vi "Get Enabled Measurements.vi"(8 "error in (no error)":errorcluster, 11 "Cluster in":T1) -> (0 "error out":errorcluster, 3 "Enabled Measurements":bool[](array[boolean]))   [LabVIEW 2019, in "ZenGage v3.0 UI.lvclass"]
uses:
  ZenGage v3.0 UI.lvclass
  <vilib>/Utility/miscctls.llb/LVRowAndColumnTypeDef.ctl
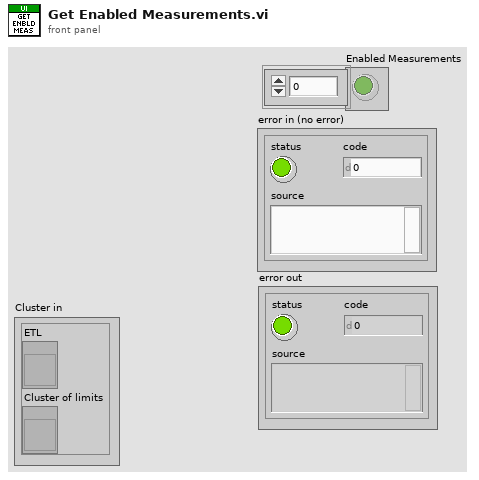
[diagram p1: front panel]
types:
  T1 = cluster{"ETL":refnum<vi>, "Cluster of limits":refnum<vi>}
  T2 = enum8{"Enabled", "Disabled", "Disabled and Grayed Out"}
  T3 = typedef "LVRowAndColumnTypeDef.ctl" = cluster{"Row":i32, "Column":i32}
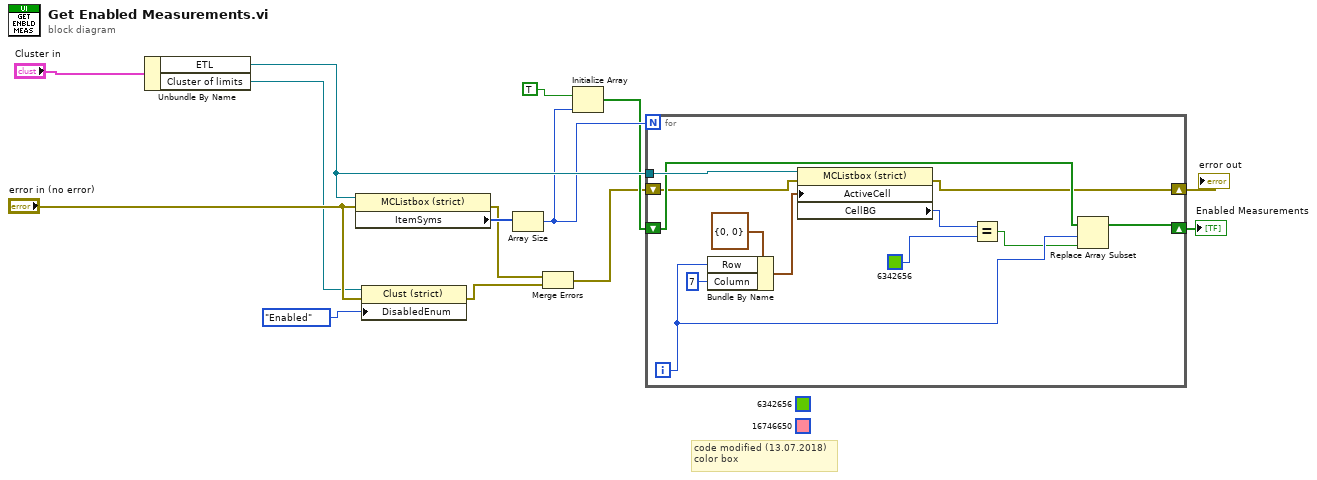
[diagram p0: block diagram]
diagram:
  (unwired) u32 6342656
  (unwired) u32 16746650
  # "code modified (13.07.2018)\ncolor box"
  n1 = Unbundle By Name("Cluster in") -> ("ETL"=w13:refnum<vi>, "Cluster of limits"=w4:refnum<vi>)
  n2 = property class="MCListbox (strict)"(reference=w13, error in="error in (no error)") -> (error out=w2:errorcluster, "ItemSyms"=w12:i32[])  [unwired: 1 out]
  n3 = property class="Clust (strict)"(reference=w4, error in="error in (no error)", "DisabledEnum"=T2."Enabled" ("Disabled")) -> (error out=w3:errorcluster)  [unwired: 1 out]
  n4 = Array Size(array=w12) -> (size(s)=w10:i32)
  n5 = Merge Errors(w2, w3) -> (w1:errorcluster)
  n6 = Initialize Array(TRUE, w10) -> (w9:bool[])
  n7 = for {
    N: w10 -> [_]
    tunnel: w13 -> [w26]
    shift-right: [w18] -> w8
    shift-left: w9 -> [w21]
    shift-right: [w16] -> w7
    shift-left: w1 -> [w17]
    i -> [w20]
    n8 = Bundle By Name(cluster=T3 {"Row"=0, "Column"=0} ("Active Cell:Active Cell"), "Row"=w20, "Column"=7) -> (w23:T3)
    n9 = property class="MCListbox (strict)"(reference=w26, error in=w17, "ActiveCell"=w23) -> (error out=w16:errorcluster, "CellBG"=w22:u32)  [unwired: 1 out]
    n10 = Equal?(x=w22, y=u32 6342656) -> (x = y?=w19:bool)
    n11 = Replace Array Subset(array=w21, new element=w19, index=w20) -> (w18:bool[])
  }
  "Enabled Measurements" <- w8
  "error out" <- w7
